vi "StringToUShort.vi"(1 "string":string) -> (0 "UShort":u16)   [LabVIEW 2009]
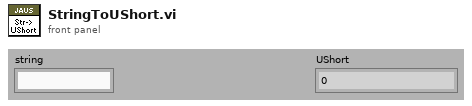
[diagram p1: front panel]
types:
  T1 = enum16{"big-endian, network order", "native, host order", "little-endian"}
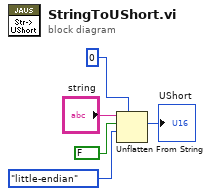
[diagram p0: block diagram]
diagram:
  n1 = Unflatten From String(type=u16 0, binary string="string", data includes array or string size? (T)=FALSE, byte order (0:big-endian, network order)=T1."little-endian") -> (value=→"UShort":u16)  [unwired: 1 in, 2 out]
